vi "Area of Triangle.vi"(1 "C边(cm)":dbl, 2 "B边(cm)":dbl, 3 "A边(cm)":dbl) -> (0 "三角形面积(cm^2)":dbl)   [LabVIEW 2012]
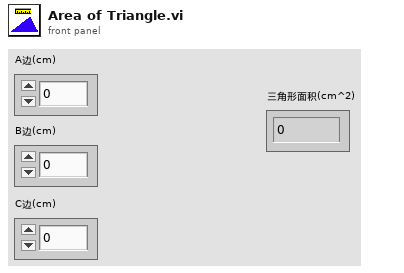
[diagram p1: front panel]
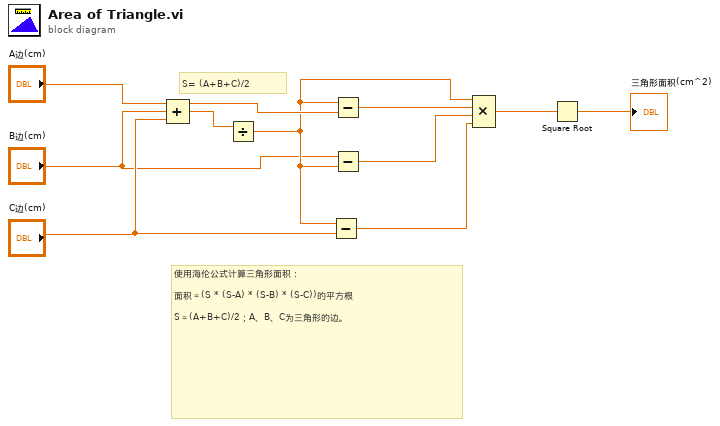
[diagram p0: block diagram]
diagram:
  # "S= (A+B+C)/2"
  # "使用海伦公式计算三角形面积：\n\n面积＝(S * (S-A) * (S-B) * (S-C))的平方根\n\nS＝(A+B+C)/2；A、B、C为三角形的边。"
  n1 = Compound Arithmetic op=ADD ("复合运算")("A边(cm)", "B边(cm)", "C边(cm)") -> (w3:dbl)
  n2 = Divide ("除")(x=w3) -> (x/y=w2:dbl)  [unwired: 1 in]
  n3 = Subtract ("减")(x=w2, y="C边(cm)") -> (x-y=w6:dbl)
  n4 = Subtract ("减")(x=w2, y="A边(cm)") -> (x-y=w8:dbl)
  n5 = Subtract ("减")(x="B边(cm)", y=w2) -> (x-y=w7:dbl)
  n6 = Compound Arithmetic op=MULTIPLY ("复合运算")(w2, w8, w7, w6) -> (w5:dbl)
  n7 = Square Root ("平方根")(x=w5) -> (sqrt(x)=→"三角形面积(cm^2)":dbl)
